vi "Measure DC Current5.vi"(8 "error in (no error)":errorcluster, 10 "measurementservice_SMUConfigResponse_Data":T1, 11 "SMUSession":refnum<k15>) -> (0 "error out":errorcluster, 1 "Compliance/Limit Reached":bool, 2 "Current Measurement":sgl, 3 "Voltage Measurement":sgl)   [LabVIEW 2019, in "HVC5.lvlib" / "HVC5.lvclass"]
doc: "Demonstrates how to use the DC Current Output Function to force an output current. This example initializes a session, configures the Output Function, Sense, Autorange, Current Level and Voltage Limit, initiates generation, waits for a specified delay, and measures the voltage and current output. This example uses Single Point source mode."
uses:
  HVC5 Class/HVC5.lvclass
  HVC5 Class/RPC Messages/measurementservice_SMUConfigResponse/measurementservice_SMUConfigResponse_Data.ctl
  HVC5 Class/RPC Messages/measurementservice_ErrorOut/measurementservice_ErrorOut_Data.ctl
  <instrlib>/niDCPower/nidcpower.llb/niDCPower Wait For Event - Event.ctl
panel:
  # "Overview: Demonstrates how to use the DC Current Output Function to force an output current.  \nThis example initializes a session, configures the Output Function, Sense, Autorange, Current Level \nand Voltage Limit, initiates generation, waits for a specified delay, and measures the voltage and \ncurrent output.  \nRequirements: NI-DCPower\nInstructions:\n1. Select the appropriate device in the Resource Name control.\n2. Configure the parameters of the DC Current signal you'd like to output.\n3. Run the VI."
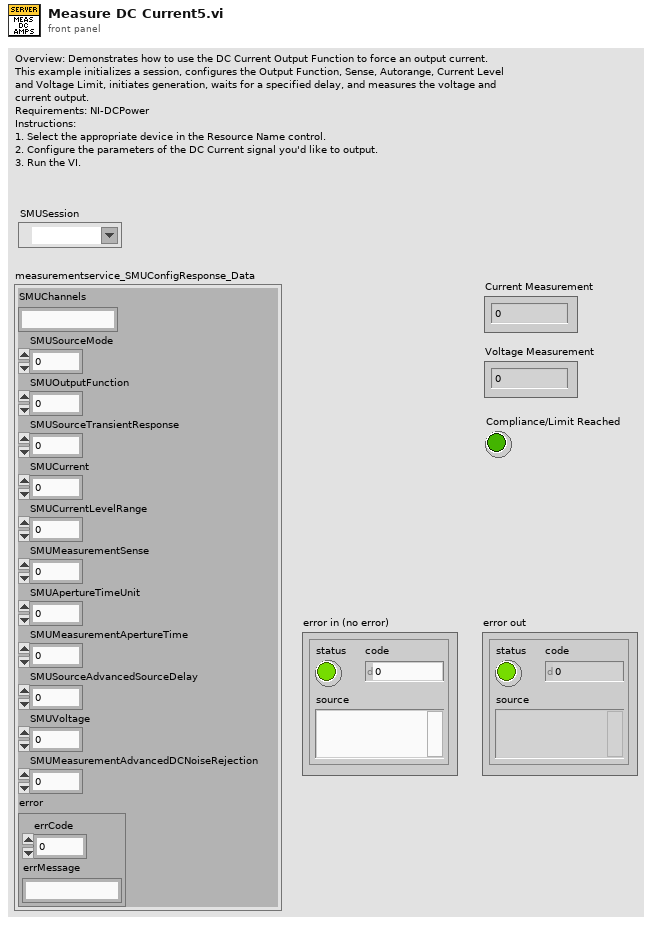
[diagram p1: front panel]
types:
  T1 = typedef "HVC5.lvlib/HVC5.lvclass/measurementservice_SMUConfigResponse_Data.ctl" = cluster{"SMUChannels":string, "SMUSourceMode":i32, "SMUOutputFunction":i32, "SMUSourceTransientResponse":i32, "SMUCurrent":sgl, "SMUCurrentLevelRange":sgl, "SMUMeasurementSense":i32, "SMUApertureTimeUnit":i32, "SMUMeasurementApertureTime":sgl, "SMUSourceAdvancedSourceDelay":sgl, "SMUVoltage":sgl, "SMUMeasurementAdvancedDCNoiseRejection":i32, "error":T2}
  T2 = typedef "HVC5.lvlib/HVC5.lvclass/measurementservice_ErrorOut_Data.ctl" = cluster{"errCode":i32, "errMessage":string}
  T3 = typedef "niDCPower Wait For Event - Event.ctl" = i32
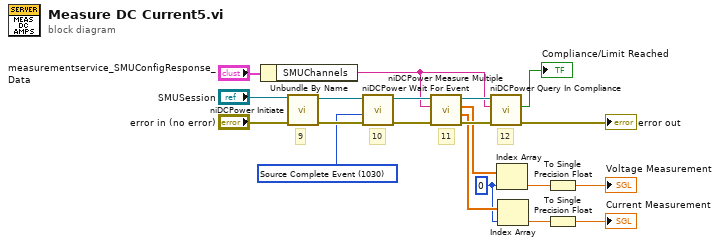
[diagram p0: block diagram]
diagram:
  w9 = T3 1030 items=["Source Complete Event"=1030, "Measure Complete Event"=1031, "Sequence Iteration Complete Event"=1032, "Sequence Engine Done Event"=1033] ("event")
  w14 = 0 ("index")
  # "11"
  # "10"
  # "12"
  # "9"
  n1 = Unbundle By Name("measurementservice_SMUConfigResponse_Data") -> ("SMUChannels"=w2:string)
  n2 = call <instrlib>:"niDCPower Initiate.vi"("error in (no error)"="error in (no error)", "instrument handle"="SMUSession") -> ("error out"=w11:errorcluster, "instrument handle out"=w13:refnum<k15>)  [unwired: 2 in, 6 out]
  n3 = call <instrlib>:"niDCPower Wait For Event.vi"("error in (no error)"=w11, "event"=w9, "instrument handle"=w13) -> ("error out"=w10:errorcluster, "instrument handle out"=w12:refnum<k15>)  [unwired: 1 in, 6 out]
  n4 = call <instrlib>:"niDCPower Measure Multiple.vi"("error in (no error)"=w10, "channel name"=w2, "instrument handle"=w12) -> ("error out"=w18:errorcluster, "current measurements"=w15:dbl[], "voltage measurements"=w16:dbl[], "instrument handle out"=w19:refnum<k15>)  [unwired: 5 out]
  n5 = call <instrlib>:"niDCPower Query In Compliance.vi"("error in (no error)"=w18, "channel name"=w2, "instrument handle"=w19) -> ("error out"=→"error out":errorcluster, "in compliance?"=→"Compliance/Limit Reached":bool)  [unwired: 7 out]
  n6 = Index Array(array=w16, index=w14) -> (element=w7:dbl)
  n7 = Index Array(array=w15, index=w14) -> (element=w5:dbl)
  n8 = To Single Precision Float(number=w7) -> (single precision float=→"Voltage Measurement":sgl)
  n9 = To Single Precision Float(number=w5) -> (single precision float=→"Current Measurement":sgl)
